vi "ReplayQueueFGV.vi"(7 "Command (ObtainQueue)":T1, 11 "PlayerName":string) -> (3 "queue out":refnum<queue>)   [LabVIEW 2015, in "ReplayBot.lvlib"]
uses:
  ReplayBot.lvlib
  TronVIEWBotAPI/MovementDirection.ctl
  ReplayQueueFGV_Command.ctl
  TronVIEWBotAPI/TronVIEWBotAPI.lvlib
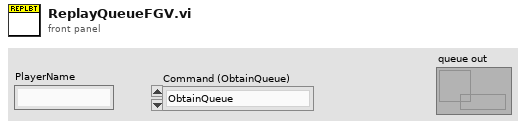
[diagram p1: front panel]
types:
  T1 = typedef "ReplayBot.lvlib/ReplayQueueFGV_Command.ctl" = enum16{"ObtainQueue", "ReleaseAllQueues"}
  T2 = typedef "TronVIEWBotAPI.lvlib/MovementDirection.ctl" = enum16{"N", "S", "W", "E"}
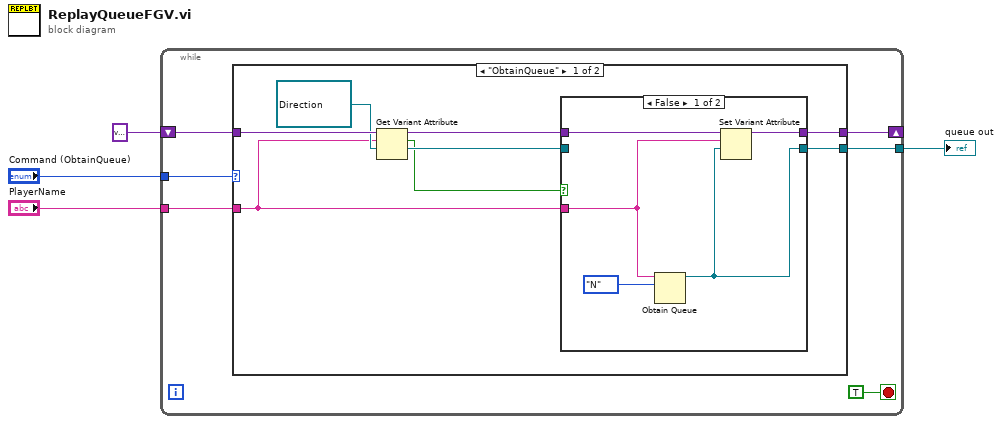
[diagram p0: block diagram]
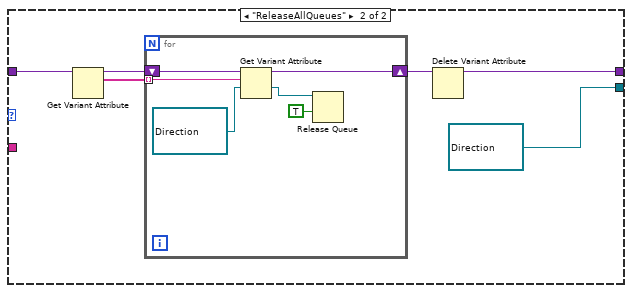
[diagram p3: hidden frame]
diagram:
  n1 = while {
    tunnel: "PlayerName" -> [w10]
    shift-right: [w6] -> _
    shift-left: variant -> [w7]
    tunnel: [w8] -> w2
    tunnel: "Command (ObtainQueue)" -> [w5]
    stop <- TRUE stop-if-true
    n2 = case shown="\"ObtainQueue\"" w5 {
      tunnel: w10 -> [w11 _]
      tunnel: [w18 w31] -> w8
      tunnel: w7 -> [w17 w30]
      tunnel: [w14 w29] -> w6
      frame "ObtainQueue" {
        w16 = refnum<queue> refnum items=["N", "S", "W", "E"] ("queue out")
        n3 = Get Variant Attribute(Variant=w17, name=w11, default value (empty Variant)=w16) -> (duplicate Variant=w15:variant, found=w12:bool, value=w13:refnum<queue>)  [unwired: 1 in, 1 out]
        n4 = case shown="False" w12 {
          tunnel: [w19 w24] -> w18
          tunnel: w15 -> [w23 w25]
          tunnel: [w21 w25] -> w14
          tunnel: w13 -> [_ w24]
          tunnel: w11 -> [w20 _]
          frame False {
            n5 = Obtain Queue(name (unnamed)=w20, element data type=MovementDirection."N" ("Direction")) -> (queue out=w19:refnum<queue>)  [unwired: 3 in, 2 out]
            n6 = Set Variant Attribute(Variant=w23, name=w20, value=w19) -> (Variant out=w21:variant)  [unwired: 1 in, 2 out]
          }
          frame True {
          }
        }
      }
      frame "ReleaseAllQueues" {
        w31 = refnum<queue> refnum items=["N", "S", "W", "E"] ("queue out")
        n7 = Get Variant Attribute(Variant=w30) -> (duplicate Variant=w28:variant, names=w26:string[])  [unwired: 3 in, 2 out]
        n8 = for {
          shift-right: [w36] -> w27
          shift-left: w28 -> [w37]
          tunnel: w26 -> [w35] mode=indexing
          w34 = refnum<queue> refnum items=["N", "S", "W", "E"] ("queue out")
          n9 = Get Variant Attribute(Variant=w37, name=w35, default value (empty Variant)=w34) -> (duplicate Variant=w36:variant, value=w33:refnum<queue>)  [unwired: 1 in, 2 out]
          n10 = Release Queue(queue=w33, force destroy? (F)=TRUE) -> ()  [unwired: 1 in, 3 out]
        }
        n11 = Delete Variant Attribute(7:w27) -> (3:w29:variant)  [unwired: 2 in, 2 out]
      }
    }
  }
  "queue out" <- w2
